vi "Change boolean text.vi"(10 "Broadcast":bool, 11 "Button Ref":refnum<vi>) -> ()   [LabVIEW 2019, in "Panther Dashboard.lvlib"]
uses:
  Panther Dashboard.lvlib
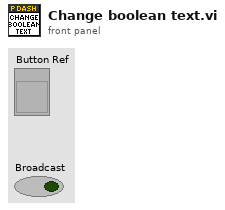
[diagram p1: front panel]
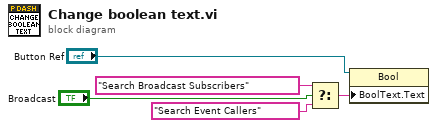
[diagram p0: block diagram]
diagram:
  n1 = Select(t="Search Broadcast Subscribers", s="Broadcast", f="Search Event Callers") -> (s? t:f=w3:string)
  n2 = property class="Bool"(reference="Button Ref", "BoolText.Text"=w3) -> ()  [unwired: 1 in, 2 out]
